vi "Read(Main).vi"(8 "error in (no error)":errorcluster, 11 "VISA resource name":refnum<visa-resource-name>) -> (0 "error out":errorcluster, 1 "Secondary Value":dbl, 2 "Primary Value":dbl, 3 "VISA resource name out":refnum<visa-resource-name>)   [LabVIEW 2014, in "LCR Meter.lvlib"]
doc: "Query the latest measurement data of the primary and secondary parameters."
uses:
  <instrlib>/LCR Meter/Examples/LCR Meter Acquire Single_1 Folder/LCR Meter.lvlib
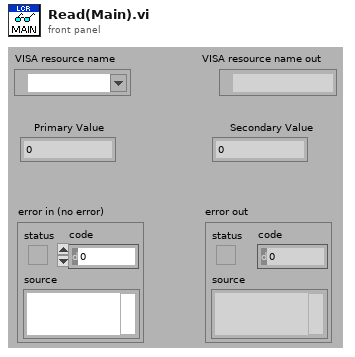
[diagram p1: front panel]
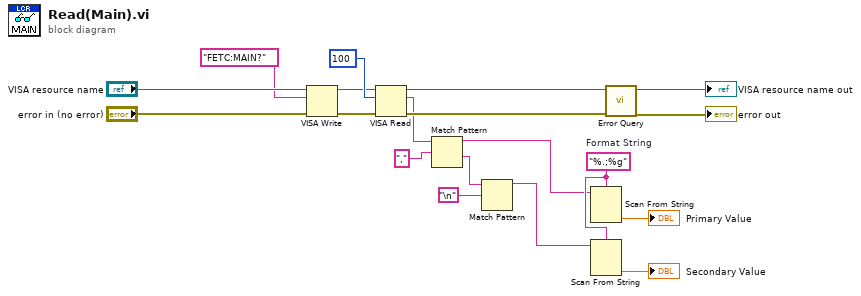
[diagram p0: block diagram]
diagram:
  w4 = "%.;%g"  # Format String
  n1 = VISA Write(VISA resource name="VISA resource name", write buffer="FETC:MAIN?", error in (no error)="error in (no error)") -> (VISA resource name out=w13:refnum<visa-resource-name>, error out=w12:errorcluster)  [unwired: 1 out]
  n2 = VISA Read(VISA resource name=w13, byte count=u32 100, error in (no error)=w12) -> (VISA resource name out=w11:refnum<visa-resource-name>, read buffer=w1:string, error out=w10:errorcluster)  [unwired: 1 out]
  n3 = Match Pattern(string=w1, regular expression=",") -> (before substring=w3:string, after substring=w8:string)  [unwired: 1 in, 2 out]
  n4 = Match Pattern(string=w8, regular expression="\n") -> (before substring=w2:string)  [unwired: 1 in, 3 out]
  n5 = Scan From String(format string=w4, input string=w3) -> (output 1=→"Primary Value":dbl)  [unwired: 3 in, 3 out]
  n6 = Scan From String(format string=w4, input string=w2) -> (output 1=→"Secondary Value":dbl)  [unwired: 3 in, 3 out]
  n7 = call <instrlib>:"Error Query.vi"("error in (no error)"=w10, "VISA resource name"=w11) -> ("error out"=→"error out":errorcluster, "VISA resource name out"=→"VISA resource name out":refnum<visa-resource-name>)  [unwired: 6 in, 2 out]
